vi "Interpolate 2D Scattered_Average.vi"(0 "X In":dbl[](array[numeric]), 5 "Y In":dbl[](array[numeric]), 7 "Z In":dbl[](array[numeric]), 9 "Xi In":dbl[](array[numeric]), 11 "Yi In":dbl[](array[numeric])) -> (4 "X Out":dbl[](array[numeric]), 6 "Y Out":dbl[](array[numeric]), 8 "Z Out":dbl[](array[numeric]), 10 "Xi Out":dbl[](array[numeric]), 15 "Yi Out":dbl[](array[numeric]))   [LabVIEW 2020, in "NI_AAL_Interpolation.lvlib"]
uses:
  <vilib>/gmath/NI_AAL_Interpolation.lvlib
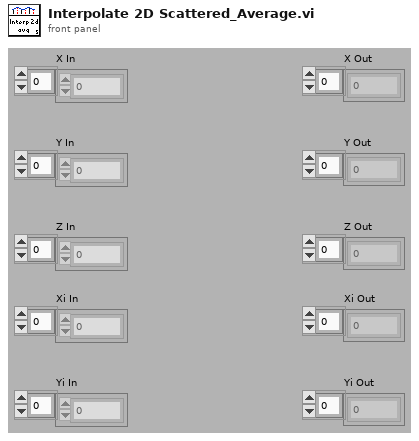
[diagram p1: front panel]
types:
  T1 = cluster{"Numeric":dbl, "Numeric":dbl, "Numeric":dbl}
  T2 = cluster{"Numeric":dbl, "Numeric":dbl, "Numeric":dbl}[]
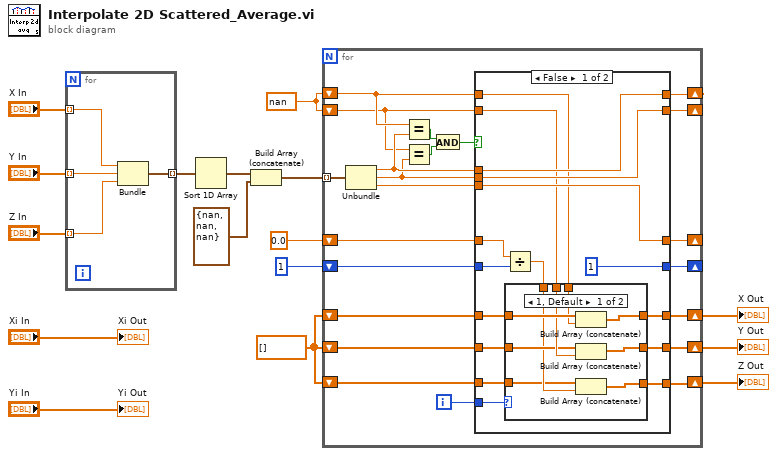
[diagram p0: block diagram]
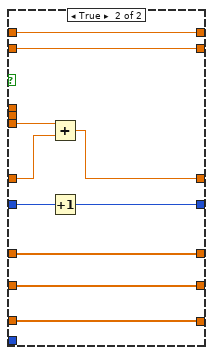
[diagram p3: hidden frame]
diagram:
  w9 = dbl[] []
  w12 = nan
  n1 = for {
    tunnel: "X In" -> [w20] mode=indexing
    tunnel: "Y In" -> [w19] mode=indexing
    tunnel: "Z In" -> [w18] mode=indexing
    tunnel: [w17] -> w13 mode=indexing
    n2 = Bundle("Numeric"=w20, "Numeric"=w19, "Numeric"=w18) -> (w17:T1)  [unwired: 1 out]
  }
  n3 = Sort 1D Array(array=w13) -> (sorted array=w5:T2)
  n4 = Build Array (concatenate)(w5, T1 {"Numeric"=nan, "Numeric"=nan, "Numeric"=nan}) -> (w4:T2)
  n5 = for {
    tunnel: w4 -> [w42] mode=indexing
    shift-right: [w30] -> _
    shift-left: w12 -> [w32]
    shift-right: [w29] -> _
    shift-left: w12 -> [w31]
    shift-right: [w35] -> _
    shift-left: 0.0 -> [w38]
    shift-right: [w27] -> _
    shift-left: 1 -> [w28]
    shift-right: [w23] -> w8
    shift-left: w9 -> [w26]
    shift-right: [w22] -> w7
    shift-left: w9 -> [w25]
    shift-right: [w21] -> w6
    shift-left: w9 -> [w24]
    i -> [w37]
    n6 = Unbundle(w42) -> ("Numeric"=w34:dbl, "Numeric"=w33:dbl, "Numeric"=w36:dbl)
    n7 = Equal?(x=w32, y=w34) -> (x = y?=w40:bool)
    n8 = Equal?(x=w31, y=w33) -> (x = y?=w41:bool)
    n9 = And(x=w40, y=w41) -> (x .and. y?=w39:bool)
    n10 = case shown="False" w39 {
      tunnel: w38 -> [w45 w79]
      tunnel: w37 -> [w54 _]
      tunnel: w36 -> [w58 w80]
      tunnel: [w58 w78] -> w35
      tunnel: w34 -> [w57 _]
      tunnel: w33 -> [w56 _]
      tunnel: w32 -> [w50 w77]
      tunnel: w31 -> [w49 w76]
      tunnel: [w57 w77] -> w30
      tunnel: [w56 w76] -> w29
      tunnel: w28 -> [w44 w75]
      tunnel: [1 w74] -> w27
      tunnel: w26 -> [w53 w73]
      tunnel: w25 -> [w52 w72]
      tunnel: w24 -> [w51 w71]
      tunnel: [w48 w73] -> w23
      tunnel: [w47 w72] -> w22
      tunnel: [w46 w71] -> w21
      frame False {
        n11 = Divide(x=w45, y=w44) -> (x/y=w43:dbl)
        n12 = case shown="1, Default" w54 {
          tunnel: w53 -> [w67 w70]
          tunnel: w52 -> [w63 w69]
          tunnel: w51 -> [w60 w68]
          tunnel: w50 -> [w66 _]
          tunnel: w49 -> [w64 _]
          tunnel: w43 -> [w61 _]
          tunnel: [w65 w70] -> w48
          tunnel: [w62 w69] -> w47
          tunnel: [w59 w68] -> w46
          frame 1, Default {
            n13 = Build Array (concatenate)(w67, w66) -> (w65:dbl[])
            n14 = Build Array (concatenate)(w63, w64) -> (w62:dbl[])
            n15 = Build Array (concatenate)(w60, w61) -> (w59:dbl[])
          }
          frame 0 {
          }
        }
      }
      frame True {
        n16 = Add(x=w80, y=w79) -> (x+y=w78:dbl)
        n17 = Increment(x=w75) -> (x+1=w74:i32)
      }
    }
  }
  "X Out" <- w8
  "Y Out" <- w7
  "Z Out" <- w6
  "Xi Out" <- "Xi In"
  "Yi Out" <- "Yi In"
